vi "sub_gmap_init.vi"(8 "error in":errorcluster, 11 "GMapControl":refnum<k24>) -> (0 "error out":errorcluster)   [LabVIEW 2019]
uses:
  C:/Users/WEGO/Documents/GitHub/Patrolrobot/Subvi/Gmap/dll/GMap.NET.WindowsForms.dll
  Patrolrobot/Subvi/Gmap/dll/GMap.NET.WindowsForms.dll
  gmap_fgv-cmd.ctl
  marker_info.ctl
  Ctrl/cmd_common.ctl
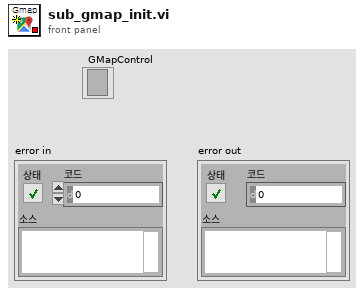
[diagram p1: front panel]
types:
  T1 = typedef "marker_info.ctl" = cluster{"arrLatLngActv":dbl[], "type":i32}
  T2 = typedef "gmap_fgv-cmd.ctl" = enum16{"marker type change", "save_image", "coll of points", "zoom n center markers", "add overlay reference", "read", "zoom", "set position by keyword", "set map provider", "map provider update", "create", "add marker", "clear marker", "close"}
  T3 = typedef "gmap_info.ctl" = cluster{"Zoon_info":cluster{"MaxZoom":dbl, "MinZoom":dbl, "Zoom":dbl}, "arrOverlayNames":string[], "MapProvider":string}
  T4 = typedef "cmd_common.ctl" = enum16{"read", "write"}
  T5 = cluster{"Lat":refnum<vi>, "Lon":refnum<vi>, "Lat_DbClk":refnum<vi>, "Lon_DbClk":refnum<vi>, "zoom":refnum<vi>, "PinDropMrkr":refnum<vi>}
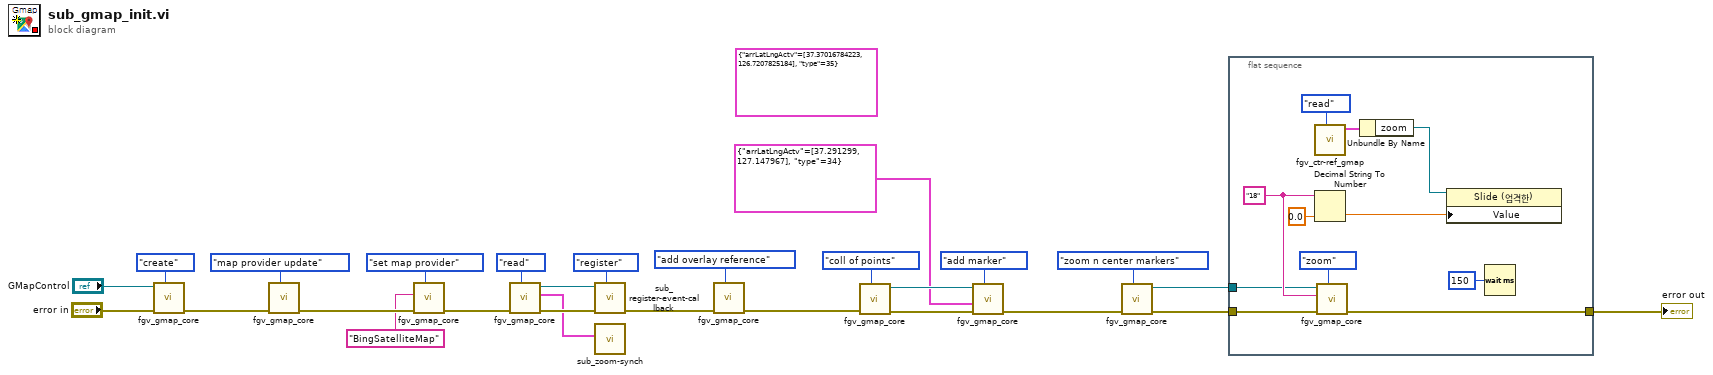
[diagram p0: block diagram]
diagram:
  (unwired) T1 {"arrLatLngActv"=[37.37016784223, 126.7207825184], "type"=35} ("marker_info")
  n1 = call "fgv_gmap_core.vi"("cmd"=gmap_fgv-cmd."create", "error in"="error in", "GMapControl"="GMapControl") -> ("error out"=w13:errorcluster)  [unwired: 5 in, 3 out]
  n2 = call "fgv_gmap_core.vi"("cmd"=gmap_fgv-cmd."map provider update", "error in"=w13) -> ("error out"=w14:errorcluster)  [unwired: 6 in, 3 out]
  n3 = call "fgv_gmap_core.vi"(7:"cmd"=gmap_fgv-cmd."set map provider" ("cmd"), "error in"=w14, 10:"cmd"="BingSatelliteMap" ("cmd")) -> ("error out"=w15:errorcluster)  [unwired: 5 in, 3 out]
  n4 = call "fgv_gmap_core.vi"("cmd"=gmap_fgv-cmd."read", "error in"=w15) -> ("error out"=w16:errorcluster, "gmap info out"=w6:T3, "GMapControl out"=w10:refnum<k24>)  [unwired: 6 in, 1 out]
  n5 = call "sub_register-event-callback.vi"("cmd"=enum16{"register", "close"}."register", "error in"=w16, "GMapControl"=w10) -> ("error out"=w11:errorcluster)  [unwired: 8 in]
  n6 = call "sub_zoom-synch.vi"("gmap info out"=w6) -> ()  [unwired: 11 in]
  n7 = call "fgv_gmap_core.vi"("cmd"=gmap_fgv-cmd."add overlay reference", "error in"=w11) -> ("error out"=w17:errorcluster)  [unwired: 6 in, 3 out]
  n8 = call "fgv_gmap_core.vi"("cmd"=gmap_fgv-cmd."coll of points", "error in"=w17) -> ("error out"=w19:errorcluster, "GMapControl out"=w20:refnum<k24>)  [unwired: 6 in, 2 out]
  n9 = call "fgv_gmap_core.vi"("cmd"=gmap_fgv-cmd."add marker", "error in"=w19, "marker_info"=T1 {"arrLatLngActv"=[37.291299, 127.147967], "type"=34}, "GMapControl"=w20) -> ("error out"=w22:errorcluster)  [unwired: 4 in, 3 out]
  n10 = call "fgv_gmap_core.vi"("cmd"=gmap_fgv-cmd."zoom n center markers", "error in"=w22) -> ("error out"=w23:errorcluster, "GMapControl out"=w24:refnum<k24>)  [unwired: 6 in, 2 out]
  n11 = flat-sequence {
    tunnel: w23 -> [w35]
    tunnel: w24 -> [w34]
    tunnel: [w32] -> w25
    frame #0 {
      w37 = "18" ("cmd")
      n12 = call "fgv_ctr-ref_gmap.vi"("cmd"=cmd_common."read") -> ("ref out"=w30:T5)  [unwired: 10 in]
      n13 = Decimal String To Number(string=w37, default (0L)=0.0 ("default (0 I32)")) -> (number=w28:dbl)  [unwired: 1 in, 1 out]
      n14 = call "fgv_gmap_core.vi"(7:"cmd"=gmap_fgv-cmd."zoom" ("cmd"), "error in"=w35, 10:"cmd"=w37, "GMapControl"=w34) -> ("error out"=w32:errorcluster)  [unwired: 4 in, 3 out]
      n15 = Unbundle By Name(w30) -> ("zoom"=w29:refnum<vi>)
      n16 = property class="Slide (엄격한)"(reference=w29, "Value"=w28) -> ()  [unwired: 1 in, 2 out]
      n17 = Wait (ms)(milliseconds to wait=u32 150) -> ()  [unwired: 1 out]
    }
  }
  "error out" <- w25
